vi "Launch Root Analog Reader.vi"(4 "Debug Alias":string, 5 "Loop Period in ms (10)":u32=10, 6 "Open Actor Core front panel? (F)":bool, 7 "DAQmx Task":refnum<k21>, 8 "error in (no error)":errorcluster, 10 "Analog Reader":refnum<class "Analog Reader.lvclass">) -> (0 "error out":errorcluster, 2 "Actor's Enqueuer":refnum<class "Message Enqueuer.lvclass">)   [LabVIEW 2024]
uses:
  Analog Reader.lvclass
  <vilib>/ActorFramework/Message Enqueuer/Message Enqueuer.lvclass
  Analog Reader.lvclass/Analog Reader.ctl
  <vilib>/ActorFramework/Actor/Actor.lvclass
  C:/Users/ottoa/OneDrive/Desktop/working copies/DAQmxActor/src/DAQmx Actor/DAQmx Actor/DAQmx Actor.lvclass
  C:/Program Files (x86)/National Instruments/LabVIEW 2024/vi.lib/ActorFramework/Actor/Actor.lvclass
  C:/Users/ottoa/OneDrive/Desktop/working copies/DAQmxActor/src/DAQmx Actor/Analog Reader/Analog Reader.lvclass
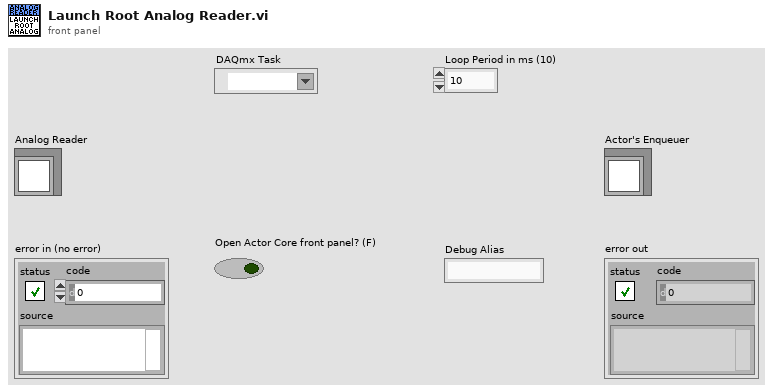
[diagram p1: front panel]
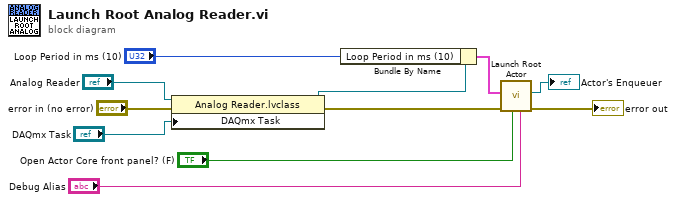
[diagram p0: block diagram]
diagram:
  n1 = property class="Analog Reader.lvclass"(reference="Analog Reader", error in="error in (no error)", "DAQmx Task"="DAQmx Task") -> (reference out=w7:refnum<class "Analog Reader.lvclass">, error out=w6:errorcluster)
  n2 = Bundle By Name(cluster=w7, "Loop Period in ms (10)"="Loop Period in ms (10)") -> (w1:cluster{})
  n3 = call <vilib>:"Launch Root Actor.vi"("Debug Alias"="Debug Alias", "Open Actor Core front panel? (F)"="Open Actor Core front panel? (F)", "error in (no error)"=w6, "Actor"=w1) -> ("error out"=→"error out":errorcluster, "Actor's Enqueuer"=→"Actor's Enqueuer":refnum<class "Message Enqueuer.lvclass">)  [unwired: 6 in]
